vi "Wire Two Objects.vi"(8 "error in (no error)":errorcluster, 10 "input cluster":T1, 11 "Data Cluster in":T2) -> (0 "error out":errorcluster, 3 "Data Cluster out":T2)   [LabVIEW 2025, in "Scripting Server.lvlib"]
uses:
  Scripting Server.lvlib
  Module Data--cluster.ctl
  Connect Objects Argument--cluster.ctl
  Connect Objects (Reply Payload)--cluster.ctl
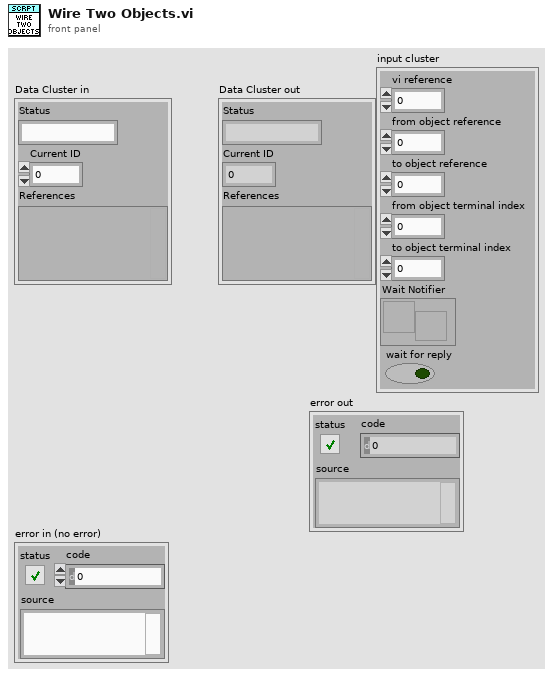
[diagram p1: front panel]
types:
  T1 = typedef "Scripting Server.lvlib/Connect Objects Argument--cluster.ctl" = cluster{"vi reference":i32, "from object reference":i32, "to object reference":i32, "from object terminal index":i32, "to object terminal index":i32, "Wait Notifier":refnum<notifier>, "wait for reply":bool}
  T2 = typedef "Scripting Server.lvlib/Module Data--cluster.ctl" = cluster{"Status":string, "Current ID":i32, "References":variant}
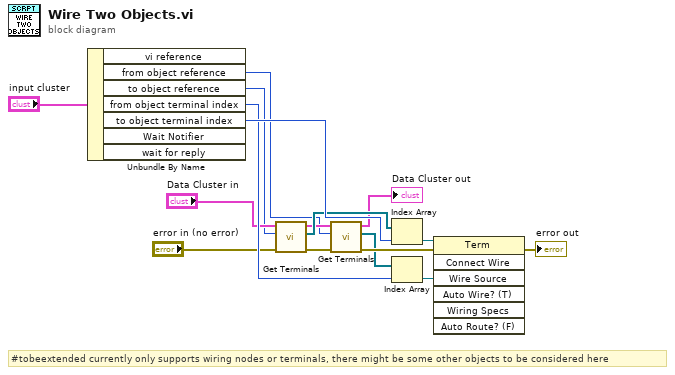
[diagram p0: block diagram]
diagram:
  # "#tobeextended currently only supports wiring nodes or terminals, there might be some other objects to be considered here"
  n1 = Unbundle By Name("input cluster") -> ("from object reference"=w4:i32, "to object reference"=w8:i32, "from object terminal index"=w12:i32, "to object terminal index"=w14:i32)  [unwired: 3 out]
  n2 = call "Get Terminals.vi"("error in (no error)"="error in (no error)", "to object reference"=w8, "Data Cluster in"="Data Cluster in") -> ("error out"=w10:errorcluster, "Terms[]"=w11:refnum<vi>[], "Data Cluster out"=w6:T2)  [unwired: 6 in]
  n3 = call "Get Terminals.vi"("error in (no error)"=w10, "to object reference"=w4, "Data Cluster in"=w6) -> ("error out"=w7:errorcluster, "Terms[]"=w3:refnum<vi>[], "Data Cluster out"=→"Data Cluster out":T2)  [unwired: 6 in]
  n4 = Index Array(array=w11, index=w14) -> (element=w13:refnum<vi>)
  n5 = Index Array(array=w3, index=w12) -> (element=w15:refnum<vi>)
  n6 = invoke class="Term" method="Connect Wire"(reference=w13, error in=w7, "Wire Source"=w15) -> (error out=→"error out":errorcluster)  [unwired: 4 in, 6 out]
